vi "HumiditySensorInput.vi"   [LabVIEW 2016]
uses:
  DHT22 - Temperature & Humidity Sensor/DHT22 Library/DHT22 (FPGA).lvlib
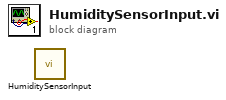
[diagram p0: block diagram]
diagram:
  n1 = call "HumiditySensorInput.vi"() -> ()  [unwired: 13 in, 3 out]
